vi "integral_ctrl.vi"(6 "Mode":T1, 8 "Sampling \nTime":dbl, 9 "Anti-windup limits":cluster{"Lower limit":dbl, "Upper limit":dbl}={"Lower limit"=-10.0, "Upper limit"=10.0}, 10 "Ti":dbl=1.0, 11 "Input":dbl) -> (0 "Sampling\nTime Out":dbl, 3 "Output":dbl)   [LabVIEW 2018, in "DiscreteControllers.lvlib"]
doc: "Integral controller implementation\nImplements: 1/(Ti*s) in discrete time.\nSelect the discretization scheme appropriately.\nAnti-windup limits can be specified as needed."
uses:
  DiscreteControllers.lvlib
  TF_diff_mode.ctl
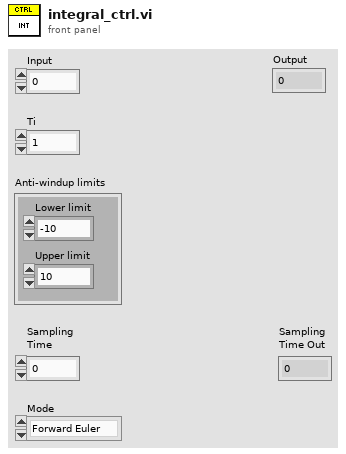
[diagram p1: front panel]
types:
  T1 = typedef "DiscreteControllers.lvlib/TF_diff_mode.ctl" = enum16{"Forward Euler", "Backward Euler", "Tustin (Bilinear)"}
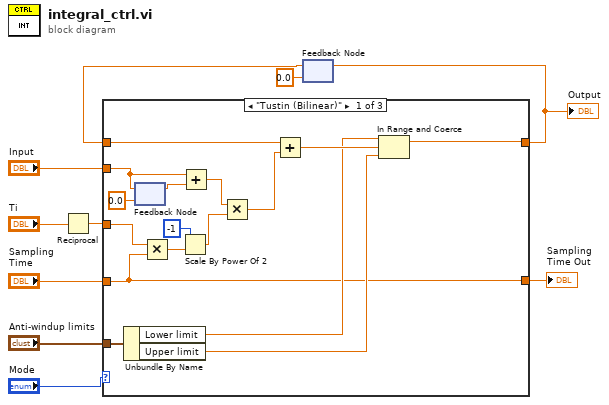
[diagram p0: block diagram]
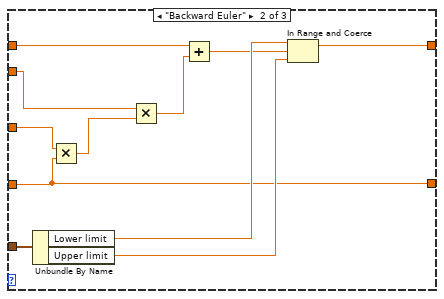
[diagram p2: hidden frame]
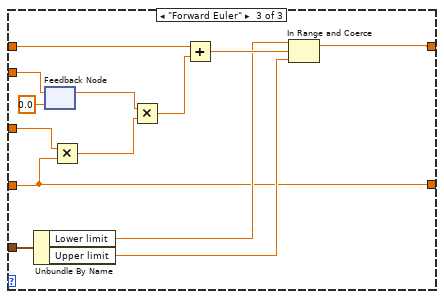
[diagram p3: hidden frame]
diagram:
  n1 = Reciprocal(x="Ti") -> (1/x=w1:dbl)
  n2 = feedback #1(0.0 ("Output")) -> (w8:dbl)
  n3 = case shown="\"Tustin (Bilinear)\"" "Mode" {
    tunnel: w8 -> [w18 w30 w45]
    tunnel: "Input" -> [w25 w29 w43]
    tunnel: w1 -> [w23 w32 w41]
    tunnel: "Sampling \nTime" -> [w11 w31 w40]
    tunnel: [w12 w33 w44] -> w5
    tunnel: "Anti-windup limits" -> [w15 w27 w38]
    tunnel: [w11 w31 w40] -> w3
    frame "Tustin (Bilinear)" {
      n4 = Unbundle By Name(w15) -> ("Lower limit"=w14:dbl, "Upper limit"=w13:dbl)
      n5 = feedback-in #2(w25) -> ()
      n6 = feedback #2(0.0 ("Input")) -> (w24:dbl)
      n7 = Multiply(x=w23, y=w11) -> (x*y=w22:dbl)
      n8 = Scale By Power Of 2(n=i16 -1, x=w22) -> (x*2^n=w19:dbl)
      n9 = Add(x=w25, y=w24) -> (x+y=w20:dbl)
      n10 = Multiply(x=w20, y=w19) -> (x*y=w17:dbl)
      n11 = Add(x=w18, y=w17) -> (x+y=w16:dbl)
      n12 = In Range and Coerce(upper limit=w14, x=w16, lower limit=w13) -> (coerced(x)=w12:dbl)  [unwired: 1 out]
    }
    frame "Backward Euler" {
      n13 = Unbundle By Name(w27) -> ("Lower limit"=w36:dbl, "Upper limit"=w37:dbl)
      n14 = Multiply(x=w32, y=w31) -> (x*y=w28:dbl)
      n15 = Multiply(x=w29, y=w28) -> (x*y=w34:dbl)
      n16 = Add(x=w30, y=w34) -> (x+y=w35:dbl)
      n17 = In Range and Coerce(upper limit=w36, x=w35, lower limit=w37) -> (coerced(x)=w33:dbl)  [unwired: 1 out]
    }
    frame "Forward Euler" {
      n18 = Unbundle By Name(w38) -> ("Lower limit"=w47:dbl, "Upper limit"=w46:dbl)
      n19 = feedback #3(0.0 ("Input")) -> (w42:dbl)
      n20 = feedback-in #3(w43) -> ()
      n21 = Multiply(x=w41, y=w40) -> (x*y=w39:dbl)
      n22 = Multiply(x=w42, y=w39) -> (x*y=w49:dbl)
      n23 = Add(x=w45, y=w49) -> (x+y=w48:dbl)
      n24 = In Range and Coerce(upper limit=w47, x=w48, lower limit=w46) -> (coerced(x)=w44:dbl)  [unwired: 1 out]
    }
  }
  "Output" <- w5
  "Sampling\nTime Out" <- w3
  n25 = feedback-in #1(w5) -> ()
